vi "GPS Data Loop With Directional Info.vi"() -> ()   [LabVIEW 2011]
panel:
  in  "GPS Data":T1
  out "GPS angle":dbl
  out "Unit Vector Long":dbl
  out "Unit Vector Lat":dbl
  out "Distance to Station":dbl
  out "Direction lat":dbl
  out "Direction long":dbl
  in  "Destination Long":dbl
  in  "Destination Lat":dbl
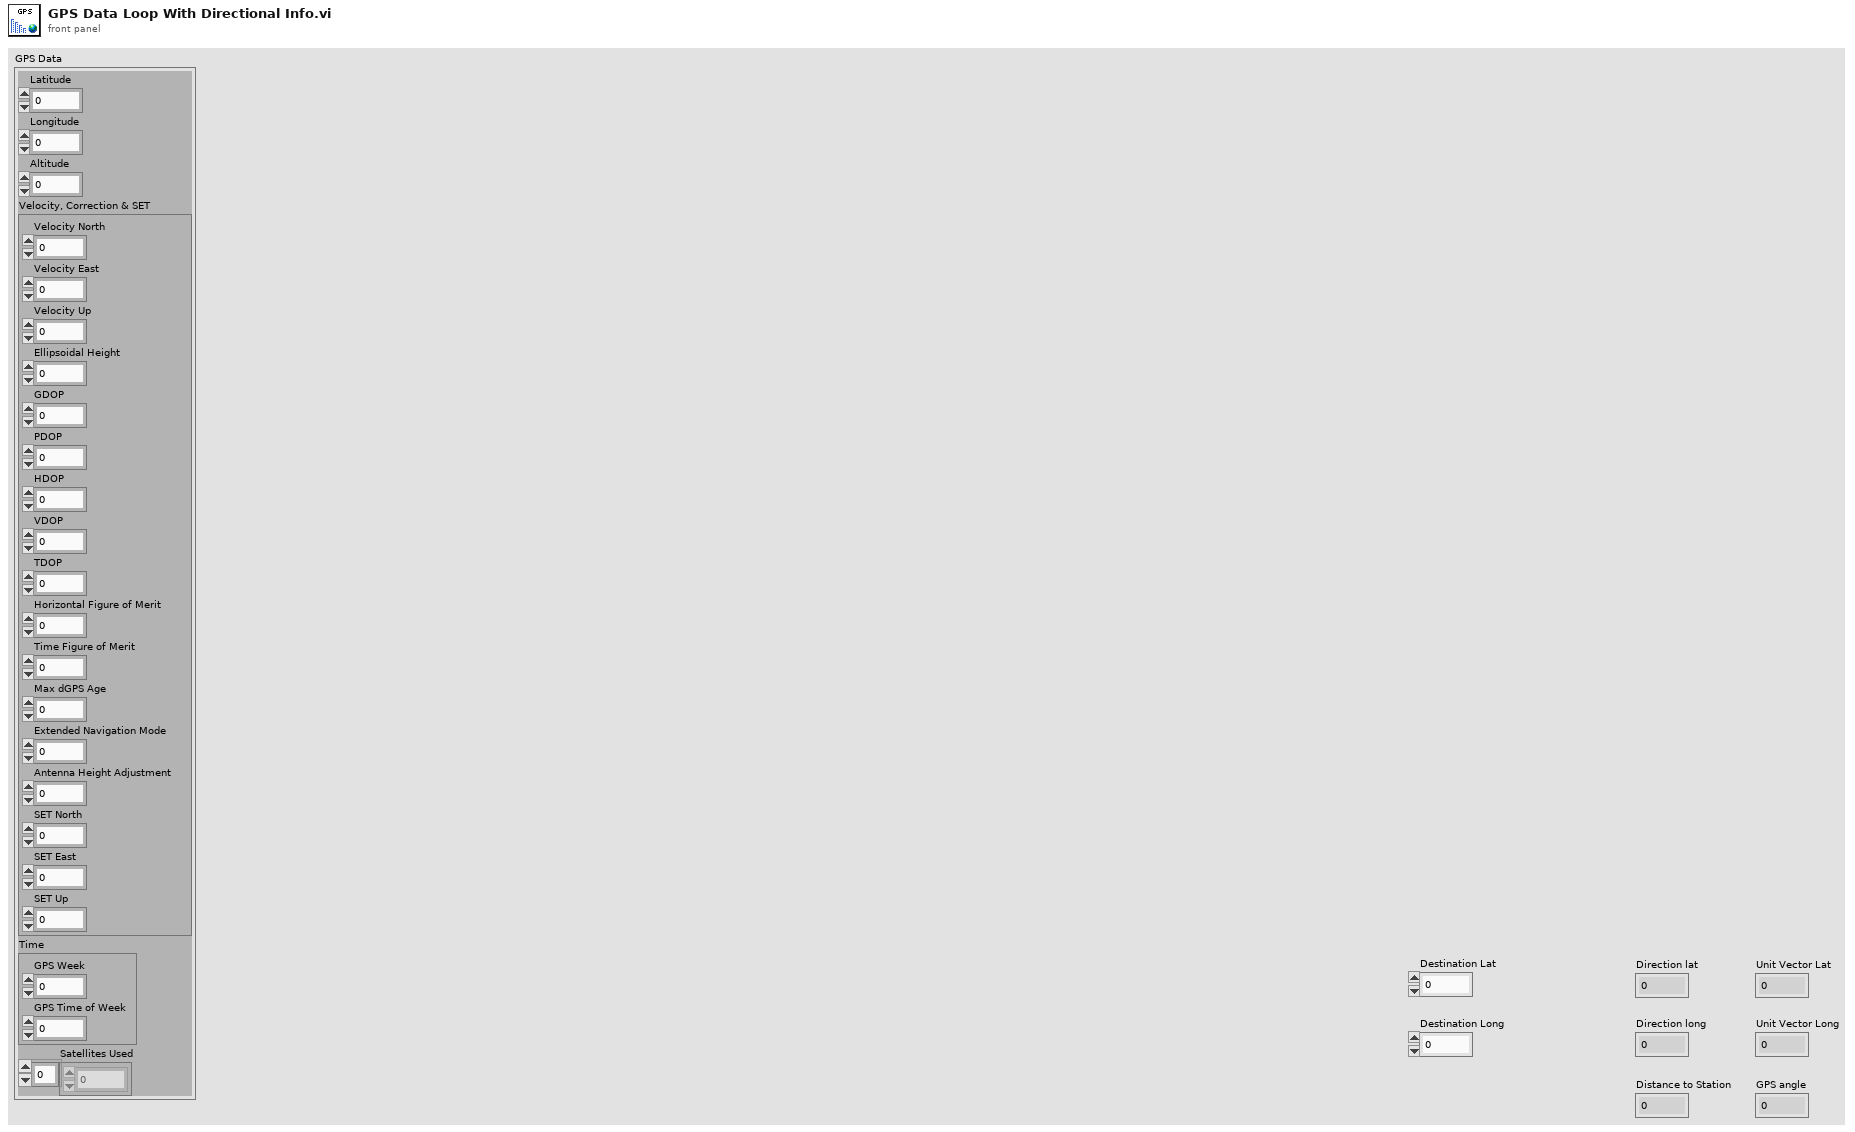
[diagram p1: front panel]
types:
  T1 = cluster{"Latitude":dbl, "Longitude":dbl, "Altitude":dbl, "Velocity, Correction & SET":cluster{"Velocity North":dbl, "Velocity East":dbl, "Velocity Up":dbl, "Ellipsoidal Height":dbl, "GDOP":sgl, "PDOP":sgl, "HDOP":sgl, "VDOP":sgl, "TDOP":sgl, "Horizontal Figure of Merit":u8, "Time Figure of Merit":u8, "Max dGPS Age":sgl, "Extended Navigation Mode":u8, "Antenna Height Adjustment ":dbl, "SET North":i32, "SET East":i32, "SET Up":i32}, "Time":cluster{"GPS Week":u16, "GPS Time of Week":sgl}, "Satellites Used":i32[]}
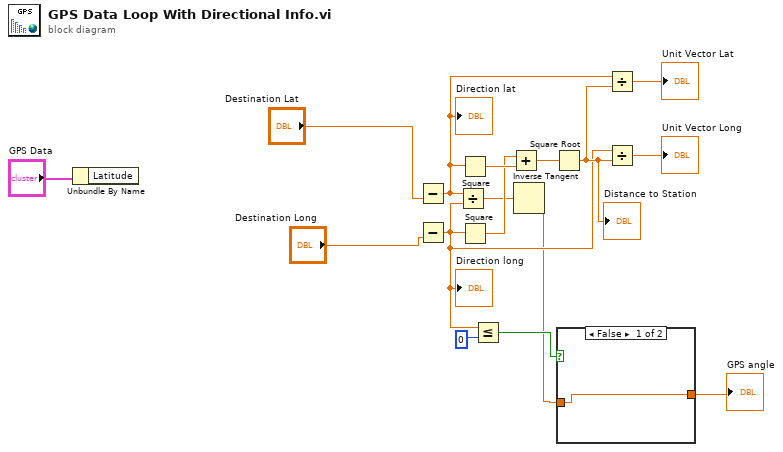
[diagram p0: block diagram]
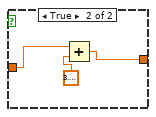
[diagram p2: hidden frame]
diagram:
  n1 = Unbundle By Name("GPS Data") -> ()  [unwired: 1 out]
  n2 = Subtract(y="Destination Lat") -> (x-y=w8:dbl)  [unwired: 1 in]
  "Direction lat" <- w8
  n3 = Subtract(y="Destination Long") -> (x-y=w5:dbl)  [unwired: 1 in]
  "Direction long" <- w5
  n4 = Divide(x=w8, y=w5) -> (x/y=w7:dbl)
  n5 = Square(x=w8) -> (x^2=w13:dbl)
  n6 = Square(x=w5) -> (x^2=w12:dbl)
  n7 = Less Or Equal?(x=w5, y=0) -> (x <= y?=w4:bool)
  n8 = Add(x=w12, y=w13) -> (x+y=w14:dbl)
  n9 = Inverse Tangent(1:w7) -> (0:w3:dbl)
  n10 = Square Root(x=w14) -> (sqrt(x)=w11:dbl)
  "Distance to Station" <- w11
  n11 = case shown="False" w4 {
    tunnel: w3 -> [w17 w19]
    tunnel: [w17 w18] -> w2
    frame False {
    }
    frame True {
      n12 = Add(x=w19, y=3.141592653589793) -> (x+y=w18:dbl)
    }
  }
  "GPS angle" <- w2
  n13 = Divide(x=w8, y=w11) -> (x/y=→"Unit Vector Lat":dbl)
  n14 = Divide(x=w5, y=w11) -> (x/y=→"Unit Vector Long":dbl)
